vi "PixelGrayUp.vi"(8 "EorIn":errorcluster, 11 "U32\nHSL-In":u32 format="%.0x") -> (0 "ErrOut":errorcluster, 3 "U32\nHSL-Out":u32 format="%.0x")   [LabVIEW 2018]
doc: "Use this template to build a VI to use as a subVI."
uses:
  <vilib>/vision/NI_Vision_Development_Module.lvlib
panel:
  # "Output Parameters"
  # "Input Parameters"
  # "VI Description:\nThis VI is .."
  # ":: MVi Framework V1.0 ::\nAuthor:Gaoke Yang\nEmail: gaoke.yang@yahoo.com\nWeb: www.mvicontrol.com\nCopyright (C) 2015, MVI Technologies All Rights Reserved"
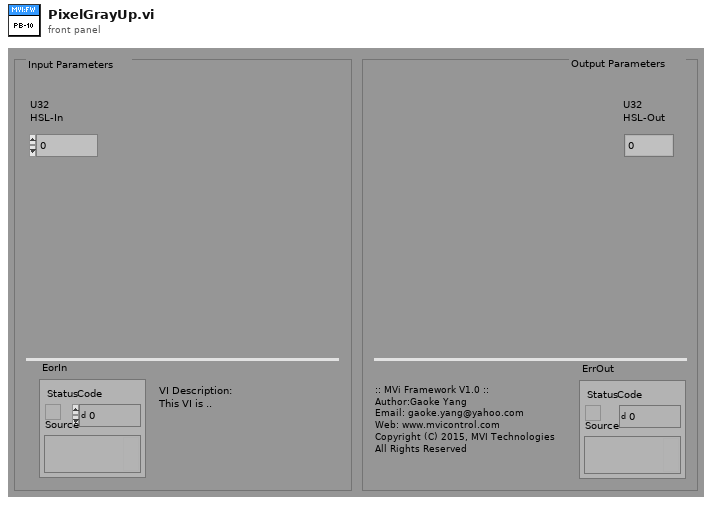
[diagram p1: front panel]
types:
  T1 = cluster{"Red (or Hue) value":u8, "Green (or Sat) value":u8, "Blue (or Light or Val) value":u8}
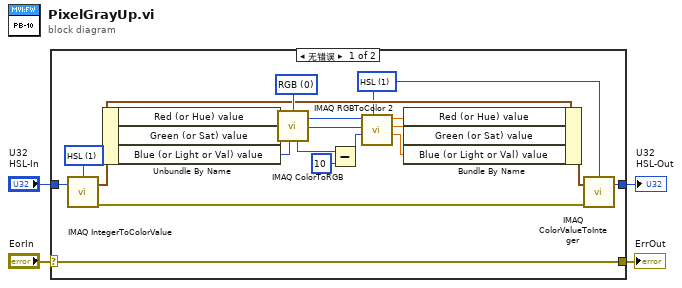
[diagram p0: block diagram]
diagram:
  n1 = case shown="无错误" "EorIn" {
    selector: "EorIn" -> [w24 w26]
    tunnel: [w24 w26] -> w3
    tunnel: "U32\nHSL-In" -> [w9 w25]
    tunnel: [w8 w25] -> w1
    frame No Error {
      w10 = u16 1 items=["RGB", "HSL", "HSV", "HSI", "CIE L*a*b*", "CIE XYZ"] ("Color Mode")
      w22 = u16 0 items=["RGB", "HSL", "HSV", "HSI"] ("Color Mode")
      w23 = u16 1 items=["RGB", "HSL", "HSV", "HSI"] ("Color Mode")
      n2 = call "IMAQ IntegerToColorValue"("U32 value"=w9, "Color Mode"=w23) -> ("error out"=w11:errorcluster, "Color Value"=w16:T1)  [unwired: 3 in, 2 out]
      n3 = Unbundle By Name(w16) -> ("Red (or Hue) value"=w21:u8, "Green (or Sat) value"=w20:u8, "Blue (or Light or Val) value"=w19:u8)
      n4 = call "IMAQ ColorToRGB"("Green or Sat value"=w20, "Blue or Luma or Val or Inten value"=w19, "Red or Hue value"=w21, "Color Mode"=w22) -> ("Blue value"=w7:u8, "Green value"=w17:u8, "Red value"=w18:u8)  [unwired: 1 in, 1 out]
      n5 = Subtract(x=w7, y=u8 10) -> (x-y=w6:u8)
      n6 = call "IMAQ RGBToColor 2"("Color Mode"=w10, "Blue value"=w6, "Green value"=w17, "Red value"=w18) -> ("Blue or Luma or Val or Inten or Z or b*value"=w13:dbl, "Green or Sat or Y or a* value"=w14:dbl, "Red or Hue or X or L* value"=w15:dbl)  [unwired: 4 in, 1 out]
      n7 = Bundle By Name(cluster=w16, "Red (or Hue) value"=w15, "Green (or Sat) value"=w14, "Blue (or Light or Val) value"=w13) -> (w12:T1)
      n8 = call "IMAQ ColorValueToInteger"("error in (no error)"=w11, "Color Value"=w12, "Color Mode"=w10) -> ("U32 value"=w8:u32)  [unwired: 2 in, 3 out]
    }
    frame Error {
    }
  }
  "ErrOut" <- w3
  "U32\nHSL-Out" <- w1
